vi "setup_variables.vi"(8 "error in (no error)":errorcluster, 9 "Variable Settings":T1={"Measurements per Iteration"=1, "Local Data Path"=path "C:/Users/Saffmanlab/Documents/Cesium/data", "Experiment description suffix for filename (no spaces please)"="", "Network Data Path"=path "Z:/", "Copy data to network"=TRUE, "Measurement Timeout (ms)"=0, "Independent Variables"=[], "Dependent Variables"=[], "Run Test Mode"=FALSE} {"Independent Variables"."# steps" min=1 step=1; "Measurements per Iteration" min=1 step=1}) -> (0 "error out":errorcluster, 3 "ExperimentVariables out":refnum<class "ExperimentVariables.lvclass">)   [LabVIEW 2012, in "ExperimentVariables.lvclass"]
uses:
  ExperimentVariables.lvclass
  Variable_Settings.ctl
  ExperimentVariables.lvclass/ExperimentVariables.ctl
panel:
  # "Parameters will be evaluated once at the beginning of the experiment from top to bottom, \nso any parameter may depend on all those above it.\nVariables will be evaluated each iteration.\nParameters and Variables may be used in various other experiment settings, as noted.\nSee LabView Help -> Formula Node and Expression Node Functions for a list of available functions."
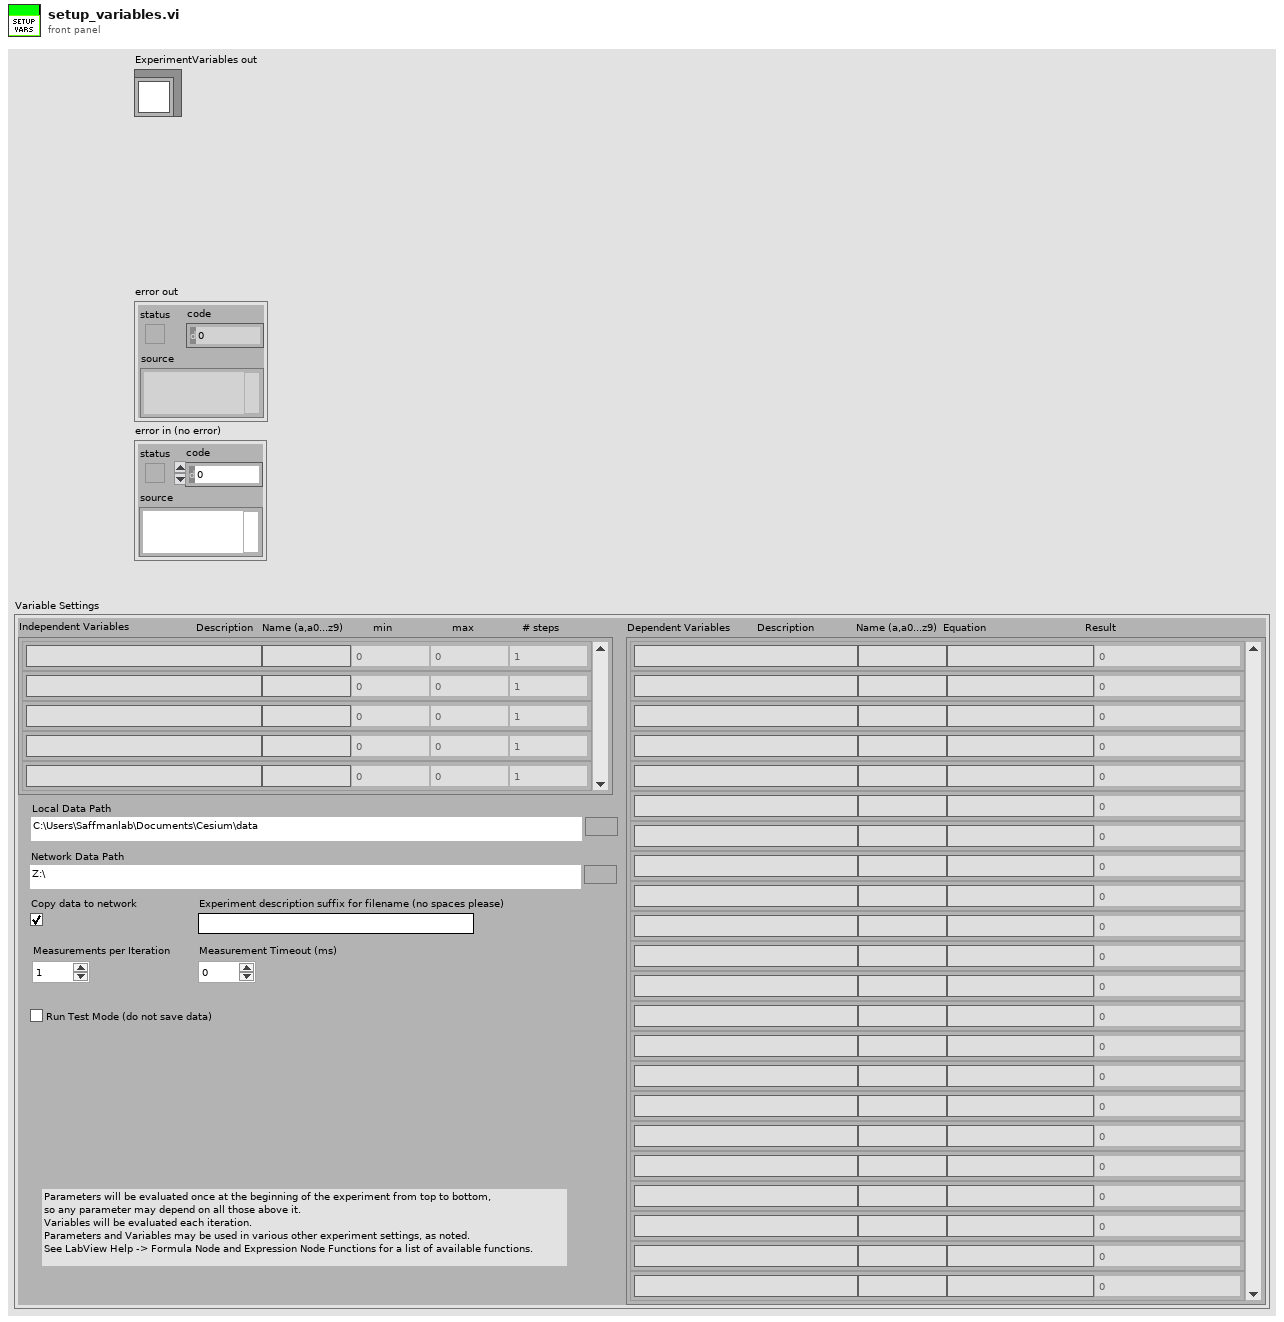
[diagram p1: front panel]
types:
  T1 = typedef "ExperimentVariables.lvclass/Variable_Settings.ctl" = cluster{"Measurements per Iteration":i32, "Local Data Path":path, "Experiment description suffix for filename (no spaces please)":string, "Network Data Path":path, "Copy data to network":bool, "Measurement Timeout (ms)":u32, "Independent Variables":cluster{"Description":string, "Name (a,a0...a9)":string, "min":dbl, "max":dbl, "# steps":u32}[], "Dependent Variables":cluster{"Description":string, "Name (a,a0...a9)":string, "Equation":string, "Result":dbl}[], "Run Test Mode":bool}
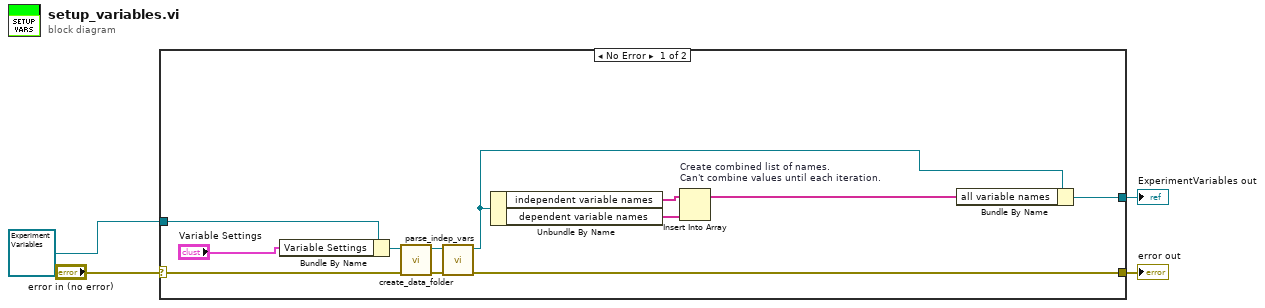
[diagram p0: block diagram]
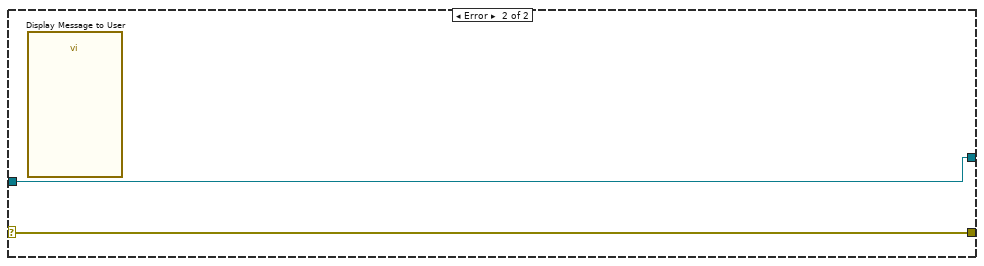
[diagram p2: hidden frame]
diagram:
  n1 = case shown="No Error" "error in (no error)" {
    selector: "error in (no error)" -> [w7 w18]
    tunnel: [w15 w18] -> w3
    tunnel: refnum<class "ExperimentVariables.lvclass"> refnum ("ExperimentVariables in") -> [w16 w17]
    tunnel: [w11 w17] -> w1
    frame No Error {
      n2 = Bundle By Name(cluster=w16, "Variable Settings"="Variable Settings") -> (w9:refnum<class "ExperimentVariables.lvclass">)
      n3 = call-dynamic "create_data_folder.vi"("error in (no error)"=w7, "ExperimentVariables in"=w9) -> ("error out"=w5:errorcluster, "ExperimentVariables out"=w6:refnum<class "ExperimentVariables.lvclass">)  [unwired: 8 in]
      n4 = call-dynamic "parse_indep_vars.vi"("error in (no error)"=w5, "ExperimentVariables in"=w6) -> ("error out"=w15:errorcluster, "ExperimentVariables out"=w12:refnum<class "ExperimentVariables.lvclass">)  [unwired: 8 in]
      n5 = Unbundle By Name(w12) -> ("independent variable names"=w14:string[], "dependent variable names"=w13:string[])
      n6 = Insert Into Array "Create combined list of names.\nCan't combine values until each iteration."(array=w14, new element=w13) -> (w10:string[])  [unwired: 1 in]
      n7 = Bundle By Name(cluster=w12, "all variable names"=w10) -> (w11:refnum<class "ExperimentVariables.lvclass">)
    }
    frame Error {
      n8 = call "Display Message to User"() -> ()  [unwired: 10 in, 2 out]
    }
  }
  "error out" <- w3
  "ExperimentVariables out" <- w1
